vi "Delete Value.vi"(8 "error in (no error)":errorcluster, 11 "pointer":i64) -> (0 "error out":errorcluster)   [LabVIEW 2024]
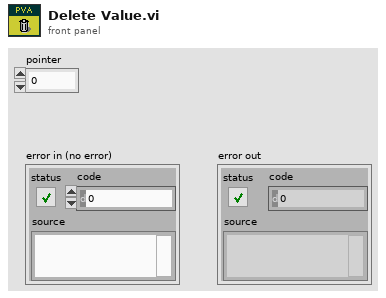
[diagram p1: front panel]
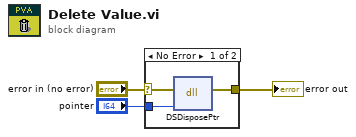
[diagram p0: block diagram]
diagram:
  n1 = case shown="No Error" "error in (no error)" {
    selector: "error in (no error)" -> [w6 w7]
    tunnel: "pointer" -> [w5 _]
    tunnel: [w4 w7] -> w1
    frame No Error {
      n2 = dll-call lib="labview" fn="DSDisposePtr"(error in=w6, "pointer"=w5) -> (error out=w4:errorcluster)  [unwired: 4 in, 1 out]
    }
    frame Error {
    }
  }
  "error out" <- w1
